vi "gfitsio-write-column-boolean-scalar.vi"(6 "row":i32, 7 "column":string, 8 "error in (no error)":errorcluster, 9 "data":bool, 11 "gfits refnum":T1) -> (0 "error out":errorcluster, 3 "dup gfits refnum":T1)   [LabVIEW 2011, in "gfitsio.lvlib"]
doc: "Write data to the table column (doing data type conversion if necessary)."
uses:
  gfitsio.lvlib
  gfitsio-refnum.ctl
  cfitsio-hdutypes.ctl
  gfitsio.dll
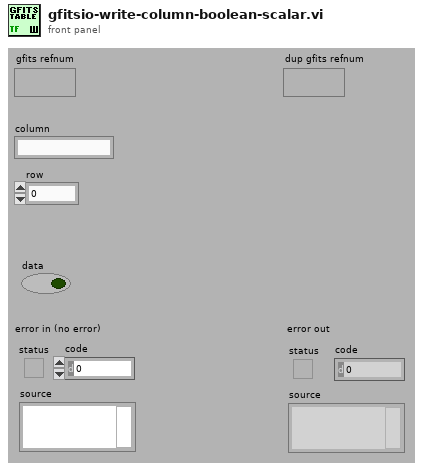
[diagram p1: front panel]
types:
  T1 = typedef "gfitsio.lvlib/gfitsio-refnum.ctl" = refnum<k1>
  T2 = typedef "gfitsio.lvlib/cfitsio-hdutypes.ctl" = i32
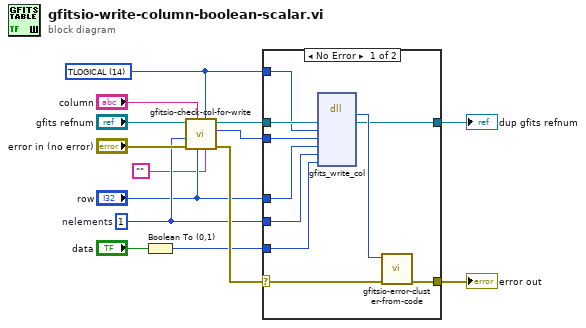
[diagram p0: block diagram]
diagram:
  w4 = T2 14 items=["TBIT"=1, "TBYTE  (U8)"=11, "TSBYTE  (I8)"=12, "TLOGICAL"=14, "TSTRING"=16, "TUSHORT  (U16)"=20, "TSHORT  (I16)"=21, "TUINT"=31, "TULONG  (U32)"=40, "TLONG  (I32)"=41, "TFLOAT  (SGL)"=42, "TLONGLONG  (I64)"=81, "TDOUBLE"=82, "TCOMPLEX  (CSG)"=83, "TDOUBLECOMPLEX  (CDB)"=163] ("cfitsio datatype")
  w5 = 1  # nelements
  n1 = Boolean To (0,1)(Boolean="data") -> (0, 1=w2:i16)
  n2 = call "gfitsio-check-col-for-write.vi"("units"="", "cfitsio datatype"=w4, "row"="row", "column"="column", "error in (no error)"="error in (no error)", "size (-1:variable)"=w5, "gfits refnum"="gfits refnum") -> ("error out"=w9:errorcluster, "colnum"=w7:i32, "dup gfits refnum"=w11:T1)  [unwired: 2 in]
  n3 = case shown="No Error" w9 {
    selector: w9 -> [w24 w26]
    tunnel: [w23 w26] -> w13
    tunnel: w11 -> [w20 w25]
    tunnel: [w21 w25] -> w14
    tunnel: w7 -> [w19 _]
    tunnel: w4 -> [w18 _]
    tunnel: "row" -> [w17 _]
    tunnel: w2 -> [w16 _]
    tunnel: w5 -> [w15 _]
    frame No Error {
      n4 = dll-call lib="C:/BonOMM/BonOMM-SAOMM/SubVIs/gfitsio/gfitsio.dll" fn="gfits_write_col"("dup gfits refnum"=w20, "datatype"=w18, "column"=w19, "row"=w17, "nelements"=w15, "data"=w16) -> (w22:i32, "dup gfits refnum"=w21:T1)  [unwired: 8 in, 2 out]
      n5 = call "gfitsio-error-cluster-from-code.vi"("error in (no error)"=w24, "error code"=w22) -> ("error out"=w23:errorcluster)  [unwired: 9 in]
    }
    frame Error {
    }
  }
  "error out" <- w13
  "dup gfits refnum" <- w14
